vi "Firing System.vi"(9 "Buttons":T2, 10 "Axes":T3, 11 "Target Info":T1(array[cluster])) -> ()   [LabVIEW 2012]
uses:
  <vilib>/Rock Robotics/WPI/Joystick/WPI_JoystickButtonState.ctl
  <vilib>/Rock Robotics/WPI/DriverStation/DriverStationLCD/WPI_DriverStationLCDLCDLine.ctl
panel:
  in  "Shooter low power":dbl(slide)=0.3 scale=0.0..1.0
  in  "Shooter high power":dbl(slide)=0.7 scale=0.0..1.0
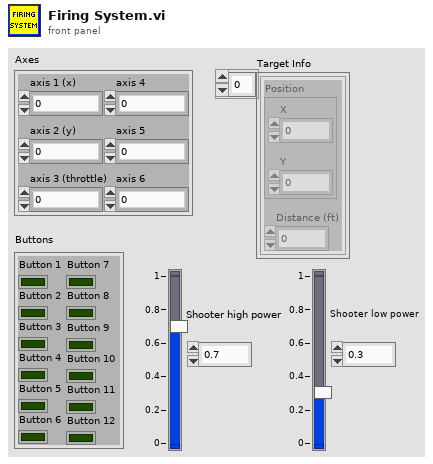
[diagram p1: front panel]
types:
  T1 = cluster{"Position":cluster{"X":dbl, "Y":dbl}, "Distance (ft)":dbl}[]
  T2 = typedef "WPI_JoystickButtonState.ctl" = cluster{"Button 1":bool, "Button 2":bool, "Button 3":bool, "Button 4":bool, "Button 5":bool, "Button 6":bool, "Button 7":bool, "Button 8":bool, "Button 9":bool, "Button 10":bool, "Button 11":bool, "Button 12":bool}
  T3 = cluster{"axis 1 (x)":dbl, "axis 2 (y)":dbl, "axis 3 (throttle)":dbl, "axis 4":dbl, "axis 5":dbl, "axis 6":dbl}
  T4 = typedef "WPI_DriverStationLCDLCDLine.ctl" = enum16{"Main - Line 1", "User - Line 2", "User - Line 3", "User - Line 4", "User - Line 5", "User - Line 6"}
  T5 = cluster{"Position":cluster{"X":dbl, "Y":dbl}, "Distance (ft)":dbl}
  T6 = typedef "WPI_MotorControlDeviceRef.ctl" = cluster{"DeviceStatus":errorcluster, "Type":enum16{"PWM", "CAN"}, "PWM":cluster{"Digital Module":T7, "PWM Channel":T8, "DeadBand":T9}, "CAN":cluster{"Device Number":u8, "Control Mode":T10, "Semaphore":T11, "Max Vout":dbl}, "Invert":bool, "TransformRef":T12, "InvTransformRef":T12}
  T7 = typedef "FPGA_TypedefDigitalModule.ctl" = enum16{"Digital Module 1", "Digital Module 2"}
  T8 = typedef "FPGA_DIOPWMChannel.ctl" = enum8{"PWM 1", "PWM 2", "PWM 3", "PWM 4", "PWM 5", "PWM 6", "PWM 7", "PWM 8", "PWM 9", "PWM 10", "Invalid"}
  T9 = typedef "WPI_PWMDeadband.ctl" = cluster{"Name":string, "maxPositivePwm":i32, "minPositivePwm":i32, "centerPwm":i32, "maxNegativePwm":i32, "minNegativePwm":i32, "angularRange":u16}
  T10 = typedef "WPI_CANJaguar_ControlMode.ctl" = enum8{"Percent VBus", "Current", "Speed", "Position", "Voltage"}
  T11 = typedef "Semaphore RefNum" = refnum<k1>
  T12 = typedef "WPI_PWMTransform_ConPane.ctl" = refnum<vi>
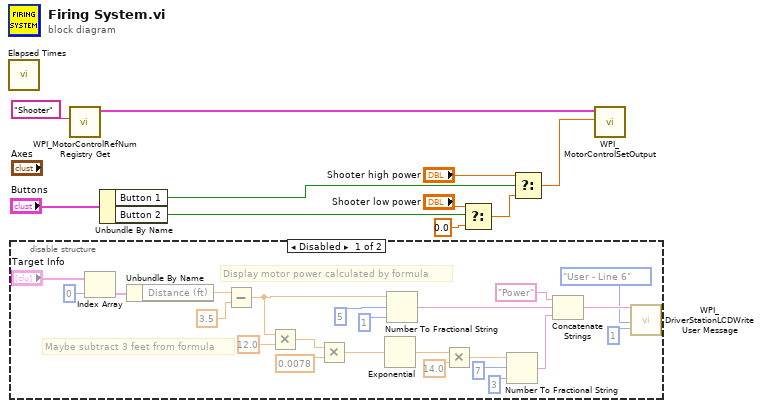
[diagram p0: block diagram]
diagram:
  n1 = call "Elapsed Times.vi"() -> ()  [unwired: 3 in, 1 out]
  n2 = disable-structure shown="Disabled" {
    frame Disabled {
      # "Maybe subtract 3 feet from formula"
      # "Display motor power calculated by formula"
      n3 = Index Array(array="Target Info", index=0) -> (element=w18:T5)
      n4 = Unbundle By Name(w18) -> ("Distance (ft)"=w13:dbl)
      n5 = Subtract(x=w13, y=3.5) -> (x-y=w12:dbl)
      n6 = Multiply(x=w12, y=12.0) -> (x*y=w32:dbl)
      n7 = Multiply(x=w32, y=0.0078) -> (x*y=w30:dbl)
      n8 = Exponential(1:w30) -> (0:w29:dbl)
      n9 = Number To Fractional String(number=w12, width (-)=i16 5, precision (6)=i16 1) -> (F-format string=w21:string)  [unwired: 1 in]
      n10 = Multiply(x=w29, y=14.0) -> (x*y=w27:dbl)
      n11 = Number To Fractional String(number=w27, width (-)=i16 7, precision (6)=i16 3) -> (F-format string=w20:string)  [unwired: 1 in]
      n12 = Concatenate Strings("Power" ("string"), w21, w20) -> (w22:string)
      n13 = call <vilib>:"WPI_DriverStationLCDWrite User Message.vi"("line text"=w22, "line"=WPI_DriverStationLCDLCDLine."User - Line 6", "starting column"=i8 1) -> ()  [unwired: 12 in, 1 out]
    }
    frame Enabled {
    }
  }
  n14 = call <vilib>:"WPI_MotorControlRefNum Registry Get.vi"("refnum name"="Shooter") -> ("MotorControlDevRef"=w9:T6)  [unwired: 9 in, 1 out]
  n15 = Unbundle By Name("Buttons") -> ("Button 1"=w6:bool, "Button 2"=w4:bool)
  n16 = Select(t="Shooter low power", s=w4, f=0.0) -> (s? t:f=w2:dbl)
  n17 = Select(t="Shooter high power", s=w6, f=w2) -> (s? t:f=w8:dbl)
  n18 = call <vilib>:"WPI_MotorControlSetOutput.vi"("Output"=w8, "MotorControlDevRef"=w9) -> ()  [unwired: 7 in, 3 out]
